vi "Create Notifiers.vi"(8 "error in (no error)":errorcluster) -> (0 "error out":errorcluster, 3 "Notifiers":T1)   [LabVIEW 2015]
uses:
  Notifires.ctl
  Notifiers.ctl
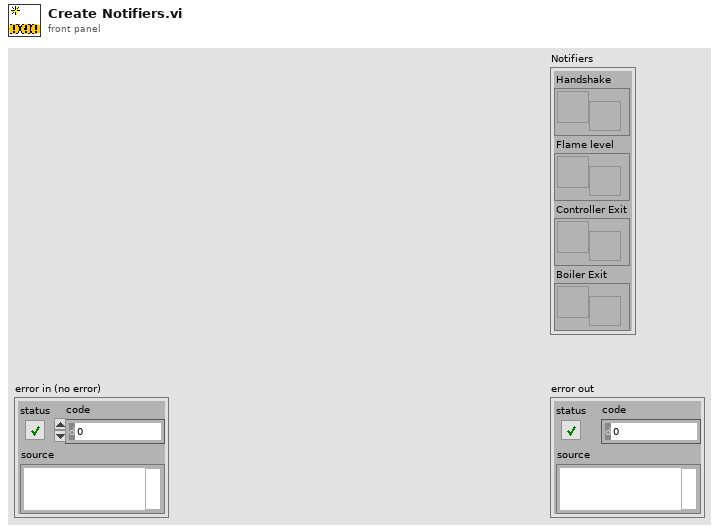
[diagram p1: front panel]
types:
  T1 = typedef "Notifires.ctl" = cluster{"Handshake":refnum<notifier>, "Flame level":T2, "Controller Exit":refnum<notifier>, "Boiler Exit":refnum<notifier>}
  T2 = typedef "Notifiers.ctl" = refnum<notifier>
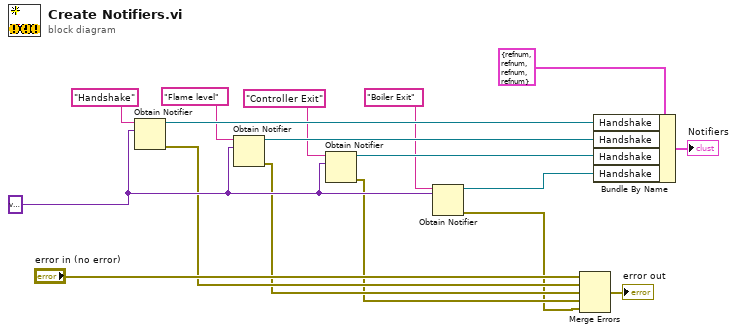
[diagram p0: block diagram]
diagram:
  w17 = variant
  n1 = Obtain Notifier(name (unnamed)="Handshake", notification data type=w17) -> (notifier out=w16:refnum<notifier>, error out=w6:errorcluster)  [unwired: 2 in, 1 out]
  n2 = Obtain Notifier(name (unnamed)="Flame level", notification data type=w17) -> (notifier out=w15:refnum<notifier>, error out=w5:errorcluster)  [unwired: 2 in, 1 out]
  n3 = Obtain Notifier(name (unnamed)="Controller Exit", notification data type=w17) -> (notifier out=w14:refnum<notifier>, error out=w4:errorcluster)  [unwired: 2 in, 1 out]
  n4 = Obtain Notifier(name (unnamed)="Boiler Exit", notification data type=w17) -> (notifier out=w13:refnum<notifier>, error out=w3:errorcluster)  [unwired: 2 in, 1 out]
  n5 = Merge Errors("error in (no error)", w6, w5, w4, w3) -> (→"error out":errorcluster)
  n6 = Bundle By Name(cluster=T1 {"Handshake"=refnum, "Flame level"=refnum, "Controller Exit"=refnum, "Boiler Exit"=refnum} ("input cluster"), "Handshake"=w16, "Handshake"=w15, "Handshake"=w14, "Handshake"=w13) -> (→"Notifiers":T1)
